vi "HandleCatch.vi"(7 "InitState":T1=enum."Catch", 8 "error in (no error)":errorcluster, 11 "Toggle?":bool) -> (0 "error out":errorcluster, 3 "State":T1=enum."Catch")   [LabVIEW 2013]
uses:
  CatchEnum.ctl
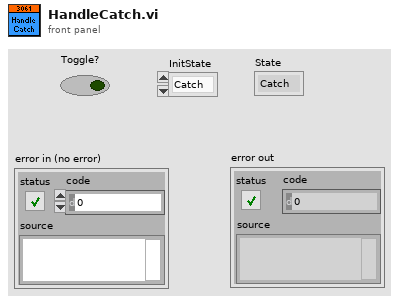
[diagram p1: front panel]
types:
  T1 = typedef "CatchEnum.ctl" = enum16{"PreCatch", "Catch", "Stop"}
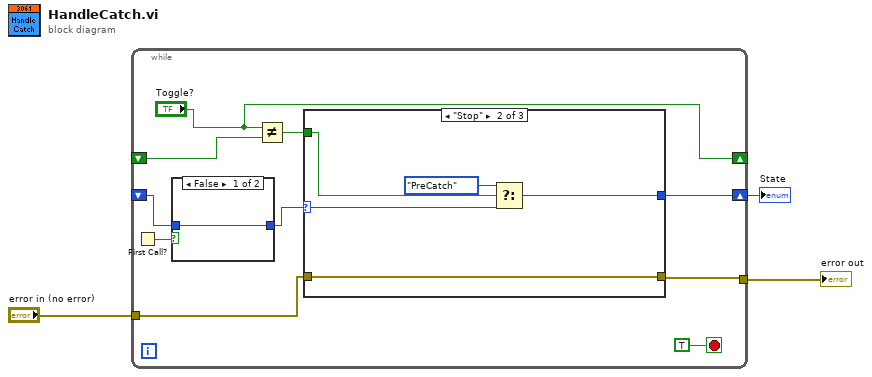
[diagram p0: block diagram]
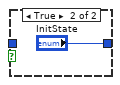
[diagram p2: hidden frame]
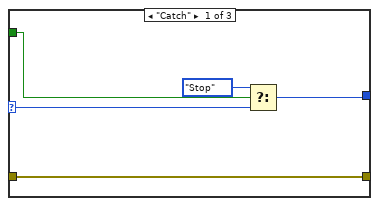
[diagram p3: hidden frame]
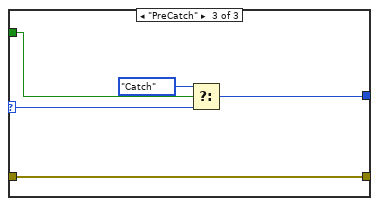
[diagram p4: hidden frame]
diagram:
  n1 = while {
    shift-right: ["Toggle?"] -> _
    shift-left: _ -> [w9]
    tunnel: "error in (no error)" -> [w11]
    tunnel: [w10] -> w2
    shift-right: [w5] -> w1
    shift-left: _ -> [w4]
    stop <- TRUE stop-if-true
    n2 = First Call?() -> (First Call?: T/F=w12:bool)
    n3 = case shown="False" w12 {
      tunnel: [w14 "InitState"] -> w6
      tunnel: w4 -> [w14 _]
      frame False {
      }
      frame True {
      }
    }
    n4 = Not Equal?(x="Toggle?", y=w9) -> (x != y?=w8:bool)
    n5 = case shown="\"Stop\"" w6 {
      selector: w6 -> [w20 w24 w30]
      tunnel: w11 -> [w19 w25 w26]
      tunnel: [w19 w25 w26] -> w10
      tunnel: w8 -> [w18 w22 w29]
      tunnel: [w16 w23 w27] -> w5
      frame "Catch" {
        n6 = Select(t=CatchEnum."Stop", s=w18, f=w20) -> (s? t:f=w16:T1)
      }
      frame "Stop" {
        n7 = Select(t=CatchEnum."PreCatch", s=w22, f=w24) -> (s? t:f=w23:T1)
      }
      frame "PreCatch" {
        n8 = Select(t=CatchEnum."Catch", s=w29, f=w30) -> (s? t:f=w27:T1)
      }
    }
  }
  "error out" <- w2
  "State" <- w1
